vi "select_mask.vi"(8 "Error In":errorcluster, 10 "Sample":string, 11 "File Path":path) -> (0 "Error Out":errorcluster)   [LabVIEW 2019]
uses:
  parameters_cluster_typedef.ctl
  select_mask_states_enum_typedef.ctl
  xi_angles_enum_typedef.ctl
  <vilib>/vision/NI_Vision_Development_Module.lvlib
panel:
  in  "Parameters":T1
  in  "Frame":i32(slide) scale=0.0..10.0
  in  "Enhance Value":sgl format="%.2f"
  in  "Enhance":T2(ring)
  in  "Next":bool
  out "Section":T3(plugin-control)
  # "Select Mask"
  # "The circle drawn indicates the approximate valid area of the sample. Create a closed contour for this sample\nin which to analyze the images. Select Next when done until all samples to be analyzed have masks set."
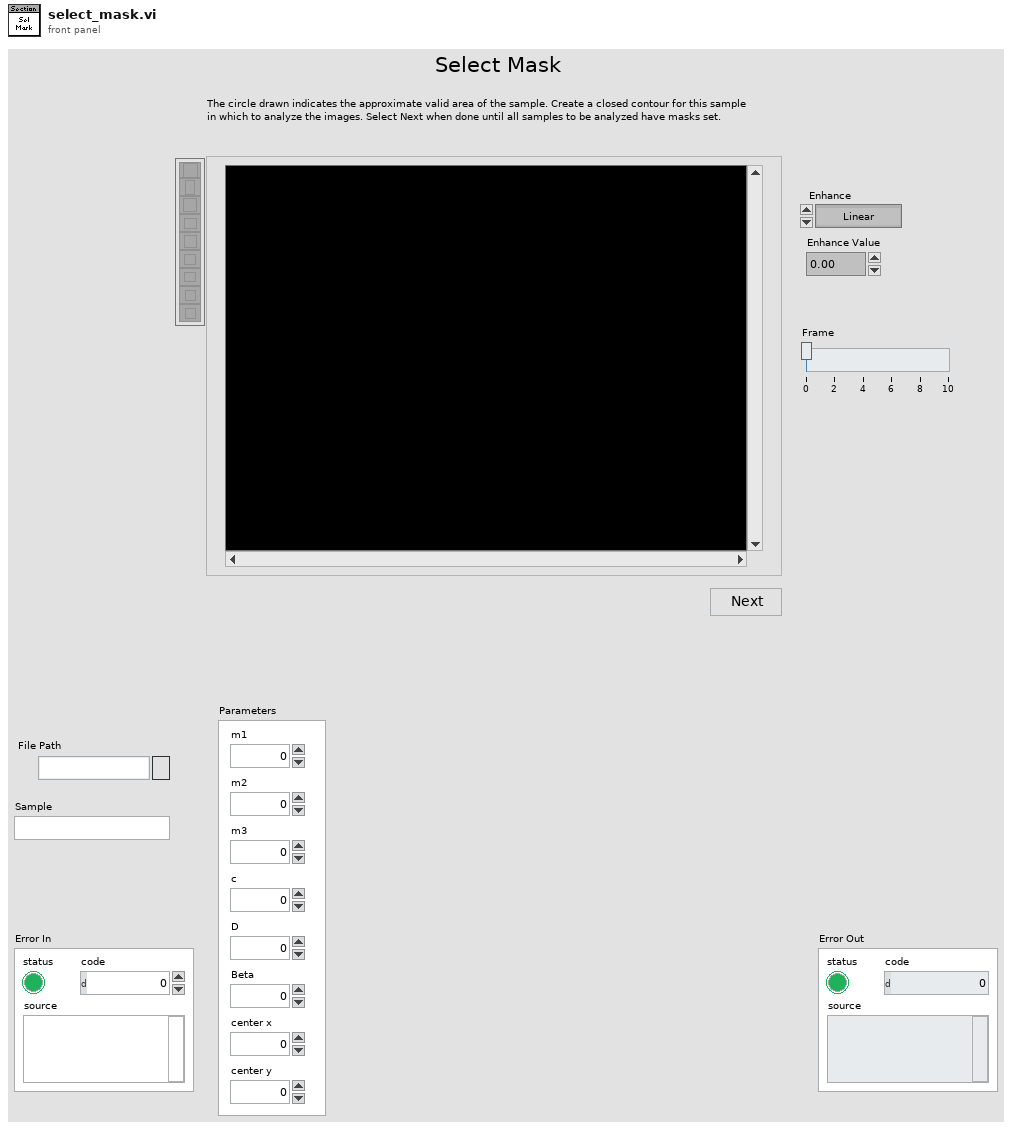
[diagram p1: front panel]
types:
  T1 = typedef "parameters_cluster_typedef.ctl" = cluster{"m1":dbl, "m2":dbl, "m3":dbl, "c":dbl, "D":dbl, "Beta":dbl, "center x":dbl, "center y":dbl}
  T2 = enum32{"Linear", "Log", "Exp", "Square", "Square root", "Power X", "Power 1/X"}
  T3 = typedef "IMAQ Image.ctl" = refnum<image>
  T4 = typedef "select_mask_states_enum_typedef.ctl" = enum16{"Shutdown", "Wait", "Plot Image", "Initialize"}
  T5 = enum16{"open", "replace", "create", "open or create", "replace or create", "replace or create with confirmation"}
  T6 = typedef "xi_angles_enum_typedef.ctl" = enum16{"0", "45"}
  T7 = cluster{"Global Rectangle":i32[], "Contours":cluster{"Contour Type":u32, "ROI Type":u32, "Points":i32[]}[]}
  T8 = cluster{"Contour Type":u32, "ROI Type":u32, "Points":i32[]}[]
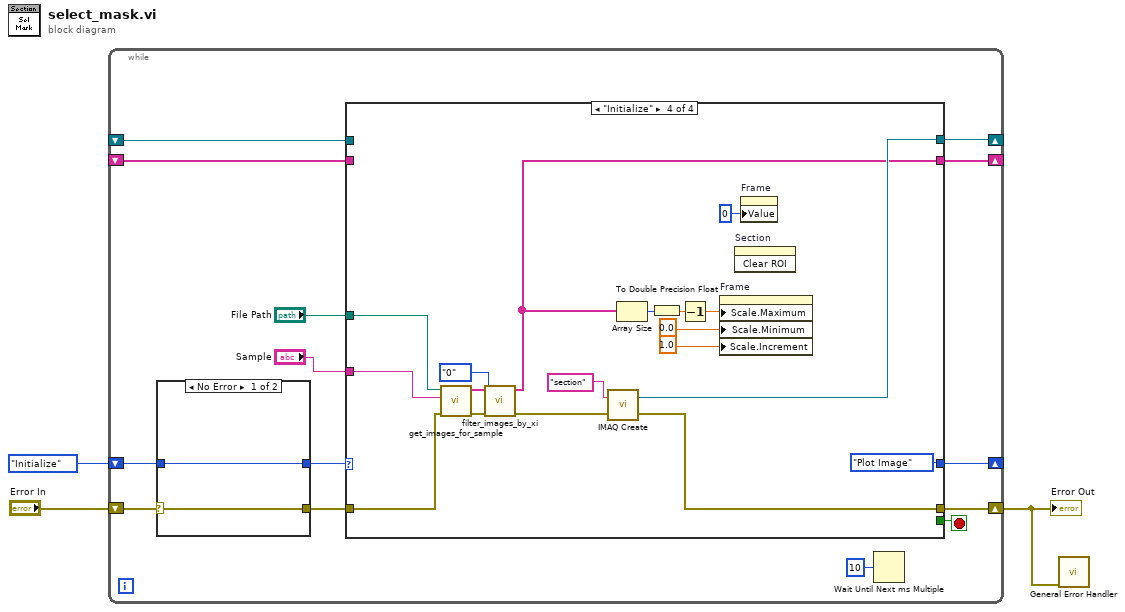
[diagram p0: block diagram]
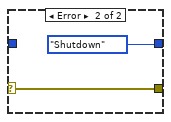
[diagram p2: hidden frame]
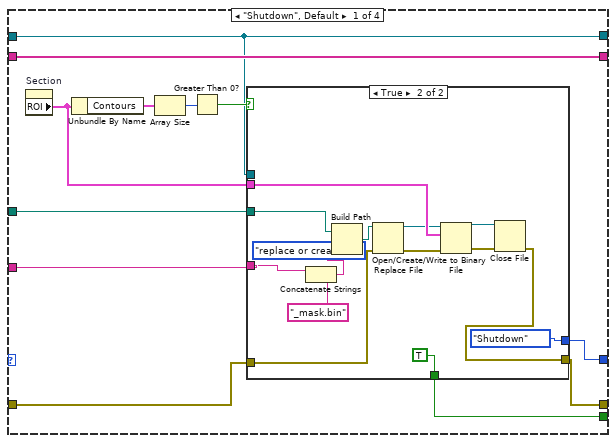
[diagram p3: hidden frame]
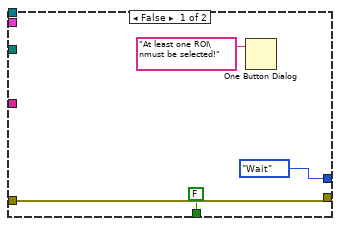
[diagram p4: hidden frame]
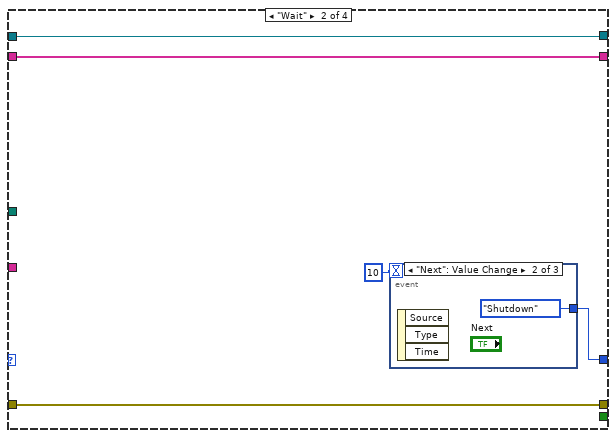
[diagram p5: hidden frame]
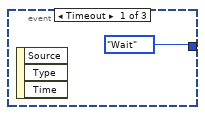
[diagram p6: hidden frame]
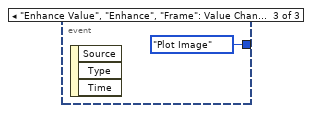
[diagram p7: hidden frame]
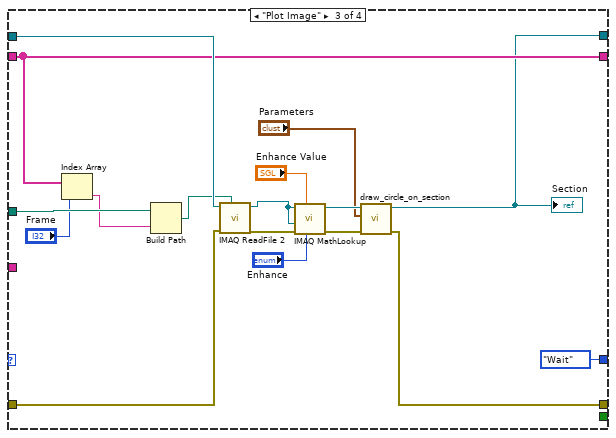
[diagram p8: hidden frame]
diagram:
  n1 = while {
    shift-right: [w13] -> _
    shift-left: select_mask_states_enum_typedef."Initialize" -> [w16]
    shift-right: [w11] -> w1
    shift-left: "Error In" -> [w17]
    shift-right: [w8] -> _
    shift-left: _ -> [w6]
    shift-right: [w7] -> _
    shift-left: _ -> [w5]
    stop <- w4 stop-if-true
    n2 = case shown="No Error" w17 {
      selector: w17 -> [w18 w21]
      tunnel: [w19 select_mask_states_enum_typedef."Shutdown"] -> w15
      tunnel: w16 -> [w19 _]
      tunnel: [w18 w21] -> w14
      frame No Error {
      }
      frame Error {
      }
    }
    n3 = case shown="\"Initialize\"" w15 {
      tunnel: w14 -> [w24 w53 w70 w87]
      tunnel: [w29 w57 select_mask_states_enum_typedef."Wait" select_mask_states_enum_typedef."Plot Image"] -> w13
      tunnel: [w23 w53 w61 w86] -> w11
      tunnel: "File Path" -> [w26 _ w74 w90]
      tunnel: "Sample" -> [w25 _ _ w89]
      tunnel: [w28 w55 w62 w88] -> w8
      tunnel: [w33 w54 w66 w80] -> w7
      tunnel: w6 -> [w28 w55 w71 _]
      tunnel: w5 -> [w33 w54 w66 _]
      tunnel: [w22 _ _ _] -> w4
      frame "Shutdown", Default {
        n4 = property on="Section" class="ImageControl"() -> ("ROI"=w27:T7)  [unwired: 2 in, 2 out]
        n5 = Unbundle By Name(w27) -> ("Contours"=w32:T8)
        n6 = Array Size(array=w32) -> (size(s)=w31:i32)
        n7 = Greater Than 0?(x=w31) -> (x > 0?=w30:bool)
        n8 = case shown="True" w30 {
          tunnel: [select_mask_states_enum_typedef."Wait" select_mask_states_enum_typedef."Shutdown"] -> w29
          tunnel: w28 -> [_ _]
          tunnel: w27 -> [_ w51]
          tunnel: w26 -> [_ w47]
          tunnel: w25 -> [_ w46]
          tunnel: w24 -> [w35 w43]
          tunnel: [w35 w38] -> w23
          tunnel: [FALSE TRUE] -> w22
          frame False {
            n9 = One Button Dialog(message="At least one ROI\nmust be selected!") -> ()  [unwired: 1 in, 1 out]
          }
          frame True {
            n10 = Concatenate Strings(w46, "_mask.bin" ("string")) -> (w44:string)
            n11 = Build Path(base path=w47, name or relative path=w44) -> (appended path=w48:path)
            n12 = Open/Create/Replace File(file path (use dialog)=w48, error in=w43, operation (0:open)=T5."replace or create") -> (refnum out=w50:refnum<file>, error out=w49:errorcluster)  [unwired: 3 in, 1 out]
            n13 = Write to Binary File(file (use dialog)=w50, data=w51, error in=w49) -> (refnum out=w40:refnum<file>, error out=w39:errorcluster)  [unwired: 3 in, 1 out]
            n14 = Close File(refnum=w40, error in=w39) -> (error out=w38:errorcluster)  [unwired: 1 out]
          }
        }
      }
      frame "Wait" {
        n15 = event shown="[1] \"Next\": Value Change" {
          selector: _ -> [_ _ _]
          dyn-events: _ -> [_ _ _]
          timeout: 10 -> [_ _ _]
          tunnel: [select_mask_states_enum_typedef."Wait" select_mask_states_enum_typedef."Shutdown" select_mask_states_enum_typedef."Plot Image"] -> w57
          event Timeout {
            n16 = event-data() -> ()  [unwired: 1 in, 3 out]
          }
          event "Next": Value Change {
            n17 = event-data() -> ()  [unwired: 1 in, 3 out]
          }
          event "Enhance Value", "Enhance", "Frame": Value Change {
            n18 = event-data() -> ()  [unwired: 1 in, 3 out]
          }
        }
      }
      frame "Plot Image" {
        n19 = Index Array(array=w66, index="Frame") -> (element=w72:string)
        n20 = Build Path(base path=w74, name or relative path=w72) -> (appended path=w69:path)
        n21 = call "IMAQ ReadFile 2"("File Path"=w69, "error in (no error)"=w70, "Image"=w71) -> ("error out"=w67:errorcluster, "Image Out"=w68:T3)  [unwired: 4 in, 3 out]
        n22 = call "IMAQ MathLookup"("Operator"="Enhance", "X Value"="Enhance Value", "error in (no error)"=w67, "Image Dst"=w68, "Image Src"=w68) -> ("error out"=w64:errorcluster, "Image Dst Out"=w65:T3)  [unwired: 5 in]
        n23 = call "draw_circle_on_section.vi"("Error In"=w64, "Parameters"="Parameters", "Image Src"=w65) -> ("Error Out"=w61:errorcluster, "Image Dst Out"=w62:T3)  [unwired: 7 in]
        "Section" <- w62
      }
      frame "Initialize" {
        n24 = call "get_images_for_sample.vi"("Error In"=w87, "Sample"=w89, "File Path"=w90) -> ("Error Out"=w81:errorcluster, "Image Names"=w83:string[])  [unwired: 7 in]
        n25 = call "filter_images_by_xi.vi"("Error In"=w81, "Xi"=xi_angles_enum_typedef."0", "Image Names"=w83) -> ("Error Out"=w79:errorcluster, "Filtered Image Names"=w80:string[])  [unwired: 7 in]
        n26 = call "IMAQ Create"("Image Name"="section", "error in (no error)"=w79) -> ("New Image"=w88:T3, "error out"=w86:errorcluster)  [unwired: 3 in]
        n27 = Array Size(array=w80) -> (size(s)=w94:i32)
        n28 = To Double Precision Float(number=w94) -> (double precision float=w84:dbl)
        n29 = Decrement(x=w84) -> (x-1=w85:dbl)
        n30 = property on="Frame" class="Slide (strict)"("Scale.Maximum"=w85, "Scale.Minimum"=0.0 ("Scale.Range:Minimum"), "Scale.Increment"=1.0 ("Scale.Range:Increment")) -> ()  [unwired: 2 in, 2 out]
        n31 = invoke on="Section" class="ImageControl" method="Clear ROI"() -> ()  [unwired: 3 in, 3 out]
        n32 = property on="Frame" class="Slide (strict)"("Value"=0 ("Frame")) -> ()  [unwired: 2 in, 2 out]
      }
    }
    n33 = Wait Until Next ms Multiple(millisecond multiple=u32 10) -> ()  [unwired: 1 out]
  }
  "Error Out" <- w1
  n34 = call <vilib>:"General Error Handler.vi"("error in (no error)"=w1) -> ()  [unwired: 10 in, 5 out]
